vi "Get Set Point Sensor Number.vi"(0 "Session Handle":T1, 11 "error in (no error)":errorcluster) -> (4 "Session Handle Out":T1, 6 "Set Point":u8, 15 "error out":errorcluster)   [LabVIEW 2015, in "Peltier.lvclass"]
uses:
  Peltier.lvclass
  Typedefs/Session Handle.ctl
  PAS/PAS.lvclass
panel:
  out "Success?":bool
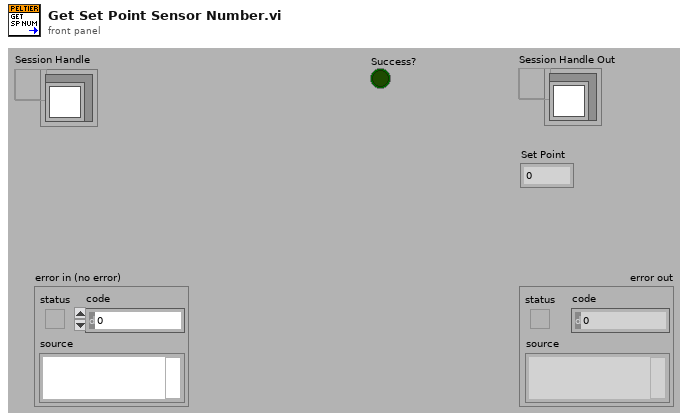
[diagram p1: front panel]
types:
  T1 = typedef "Peltier.lvclass/Session Handle.ctl" = refnum<data-value>
  T2 = typedef "XNET Frame CAN.ctl" = cluster{"timestamp":timestamp, "payload":u8[], "identifier":u32, "type":T3, "extended?":bool, "echo?":bool}
  T3 = typedef "XNET Frame Type CAN.ctl" = u8
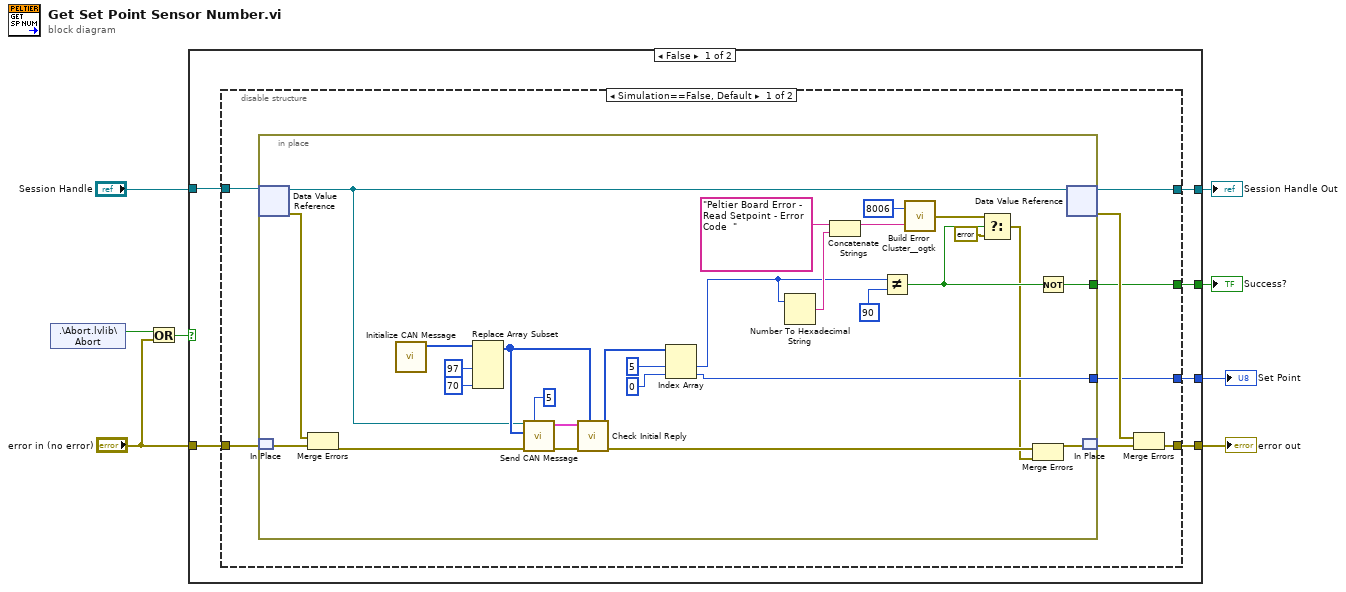
[diagram p0: block diagram]
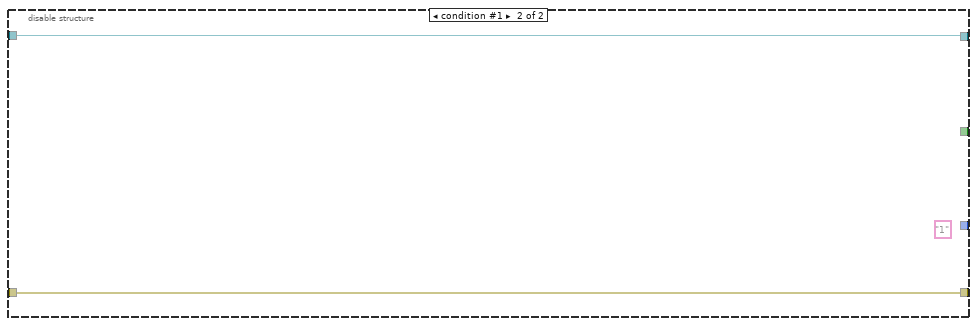
[diagram p2: hidden frame]
diagram:
  n1 = shared-variable ".\\Abort.lvlib\\Abort"() -> (w7:bool)  [unwired: 1 in, 1 out]
  n2 = Or(x=w7, y="error in (no error)") -> (x .or. y?=w5:bool)
  n3 = case shown="False" w5 {
    tunnel: [w14 w54] -> w1
    tunnel: [w13 w53] -> w8
    tunnel: "Session Handle" -> [w12 w54]
    tunnel: "error in (no error)" -> [w11 w53]
    tunnel: [w9 _] -> w4
    tunnel: [w10 _] -> w3
    frame False {
      n4 = disable-structure shown="Simulation==False, Default" {
        disable-tunnel: [w22 w52] -> w14
        disable-tunnel: [w19 w51] -> w13
        disable-tunnel: w12 -> [w18 w52]
        disable-tunnel: w11 -> [w17 w51]
        disable-tunnel: [w16 _] -> w10
        disable-tunnel: [w15 _] -> w9
        frame condition #0 (active) {
          n5 = in-place {
            in-place-border: [w32] -> w16
            in-place-border: [w26] -> w15
            n6 = in-place-dvr #1(w18) -> (w41:refnum<class "Peltier.lvclass">, w46:errorcluster)
            n7 = in-place-match #2(w17) -> (w45:errorcluster)
            n8 = Merge Errors(w46, w45) -> (w40:errorcluster)
            n9 = call "Initialize CAN Message.vi"() -> ("Initial Payload"=w48:u8[])  [unwired: 11 in]
            n10 = Replace Array Subset(array=w48, new element #1=u8 97 ("new element/subarray"), new element #2=u8 70 ("new element/subarray")) -> (w44:u8[])  [unwired: 2 in]
            n11 = call "Send CAN Message.vi"("Number of Retries"=5, "error in (no error)"=w40, "payload"=w44, "Peltier In"=w41) -> ("error out"=w25:errorcluster, "Reply"=w42:T2[])  [unwired: 5 in, 1 out]
            n12 = call "Check Initial Reply.vi"("Write Message"=w44, "error in (no error)"=w25, "Reply"=w42) -> ("error out"=w24:errorcluster, "Data Packet"=w47:u8[])  [unwired: 5 in, 2 out]
            n13 = Index Array(array=w47, index #1=5 ("index"), index #2=0 ("index")) -> (element #1=w33:u8, element #2=w26:u8)
            n14 = Number To Hexadecimal String(2:w33) -> (0:w37:string)  [unwired: 1 in]
            n15 = Concatenate Strings("Peltier Board Error -  Read Setpoint - Error Code  " ("string"), w37) -> (w36:string)
            n16 = Not Equal?(x=w33, y=u8 90 ("new element/subarray")) -> (x != y?=w28:bool)
            n17 = call <userlib>:"Build Error Cluster__ogtk.vi"("String to Prepend to source (\"\")"=w36, "code"=8006) -> ("error out"=w30:errorcluster)
            n18 = Select(t=w30, s=w28, f=errorcluster {"status"=FALSE, "code"=0, "source"=""}) -> (s? t:f=w23:errorcluster)
            n19 = Merge Errors(w24, w23) -> (w49:errorcluster)
            n20 = Not(x=w28) -> (.not. x?=w32:bool)
            n21 = in-place-dvr #1(w41) -> (w22:T1, w20:errorcluster)
            n22 = in-place-match #2(w49) -> (w21:errorcluster)
          }
          n23 = Merge Errors(w20, w21) -> (w19:errorcluster)
        }
        frame condition #1 {
          (unwired) "1"
        }
      }
    }
    frame True {
    }
  }
  "error out" <- w8
  "Set Point" <- w4
  "Success?" <- w3
  "Session Handle Out" <- w1
